vi "data2image_2d.vi"(10 "image_2d":sgl[][](array[numeric])) -> (2 "image_1d":sgl[](array[numeric]))   [LabVIEW 2014]
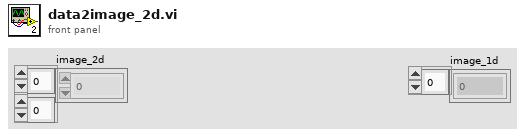
[diagram p1: front panel]
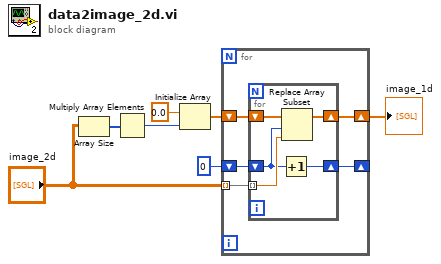
[diagram p0: block diagram]
diagram:
  n1 = Array Size(array="image_2d") -> (size(s)=w1:i32[])
  n2 = Multiply Array Elements(1:w1) -> (0:w4:i32)
  n3 = Initialize Array(sgl 0.0 ("element"), w4) -> (w6:sgl[])
  n4 = for {
    tunnel: "image_2d" -> [w12] mode=indexing
    shift-right: [w11] -> _
    shift-left: 0 -> [w10]
    shift-right: [w8] -> w3
    shift-left: w6 -> [w9]
    n5 = for {
      tunnel: w12 -> [w15] mode=indexing
      shift-right: [w17] -> w11
      shift-left: w10 -> [w14]
      shift-right: [w13] -> w8
      shift-left: w9 -> [w16]
      n6 = Increment(x=w14) -> (x+1=w17:i32)
      n7 = Replace Array Subset(array=w16, new element=w15, index=w14) -> (w13:sgl[])
    }
  }
  "image_1d" <- w3
